vi "StringStackStateMachine.vi"() -> ()   [LabVIEW 2020]
doc: "Use this template to build a queued message handler design pattern."
panel:
  out "error out":errorcluster
  in  "error in":errorcluster
  in  "stop":bool
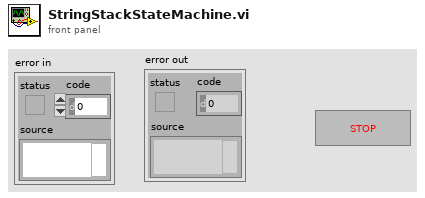
[diagram p1: front panel]
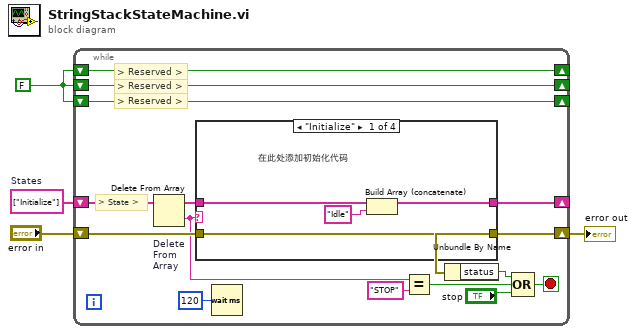
[diagram p0: block diagram]
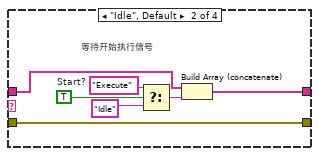
[diagram p2: hidden frame]
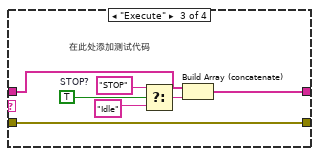
[diagram p3: hidden frame]
diagram:
  w1 = string[] ["Initialize"]  # States
  w2 = FALSE
  n1 = while {
    shift-right: [w19] -> _
    shift-left: w1 -> [w8]
    shift-right: [w13] -> w3
    shift-left: "error in" -> [w14]
    shift-right: [w11] -> _
    shift-left: w2 -> [w11]
    shift-right: [w10] -> _
    shift-left: w2 -> [w10]
    shift-right: [w9] -> _
    shift-left: w2 -> [w9]
    stop <- w16 stop-if-true
    # "> Reserved >"
    # "> Reserved >"
    # "> Reserved >"
    # "> State >"
    n2 = Delete From Array "Delete\nFrom\nArray"(array=w8) -> (deleted portion=w7:string, array with subset deleted=w6:string[])  [unwired: 2 in]
    n3 = case shown="\"Initialize\"" w7 {
      tunnel: [w20 w25 w36 w38] -> w19
      tunnel: w14 -> [w23 w30 w37 w39]
      tunnel: [w23 w30 w37 w39] -> w13
      tunnel: w6 -> [w22 w24 w31 w38]
      frame "Initialize" {
        # "在此处添加初始化代码"
        n4 = Build Array (concatenate) "Build Array"(w22, "Idle") -> (w20:string[])
      }
      frame "Idle", Default {
        w29 = TRUE  # Start?
        # "等待开始执行信号"
        n5 = Select(t="Execute", s=w29, f="Idle") -> (s? t:f=w26:string)
        n6 = Build Array (concatenate) "Build Array"(w24, w26) -> (w25:string[])
      }
      frame "Execute" {
        w35 = TRUE  # STOP?
        # "在此处添加测试代码"
        n7 = Select(t="STOP", s=w35, f="Idle") -> (s? t:f=w32:string)
        n8 = Build Array (concatenate) "Build Array"(w31, w32) -> (w36:string[])
      }
      frame "STOP" {
        # "在此处添加现场清理代码"
      }
    }
    n9 = Wait (ms)(milliseconds to wait=u32 120) -> ()  [unwired: 1 out]
    n10 = Equal?(x=w7, y="STOP") -> (x = y?=w15:bool)
    n11 = Unbundle By Name(w13) -> ("status"=w12:bool)
    n12 = Compound Arithmetic op=OR(w12, w15, "stop") -> (w16:bool)
  }
  "error out" <- w3
